vi "UI-Set Dock Button Value.vi"(8 "Error In":errorcluster, 10 "Value (F)":bool, 11 "Appearance Actor in":refnum<class "Appearance Actor.lvclass">) -> (0 "Error Out":errorcluster, 3 "Appearance Actor out":refnum<class "Appearance Actor.lvclass">)   [LabVIEW 2021, in "Appearance Actor.lvlib" / "Appearance Actor.lvclass"]
uses:
  Appearance Actor.lvclass
  Appearance Actor.lvclass/Appearance Actor.ctl
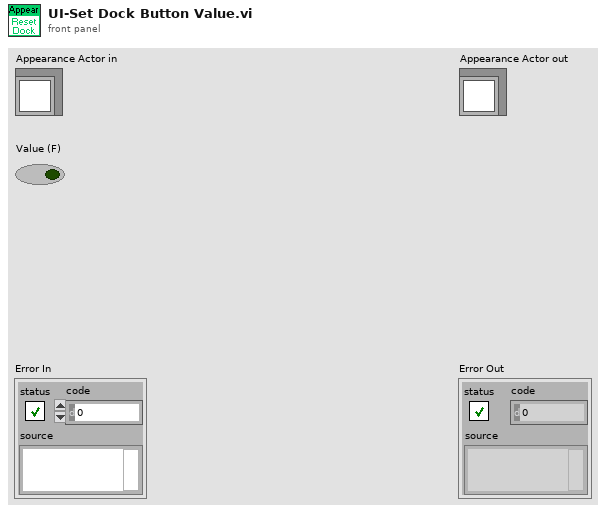
[diagram p1: front panel]
types:
  T1 = typedef "Appearance Actor.lvlib/Appearance Actor.lvclass/UI Controls--map.ctl" = map{string, T2}
  T2 = typedef "Appearance Actor.lvlib/Appearance Actor.lvclass/Element Controls--map.ctl" = map{string, T3}
  T3 = typedef "Appearance Actor.lvlib/Appearance Actor.lvclass/Controls--map.ctl" = map{string, refnum<vi>}
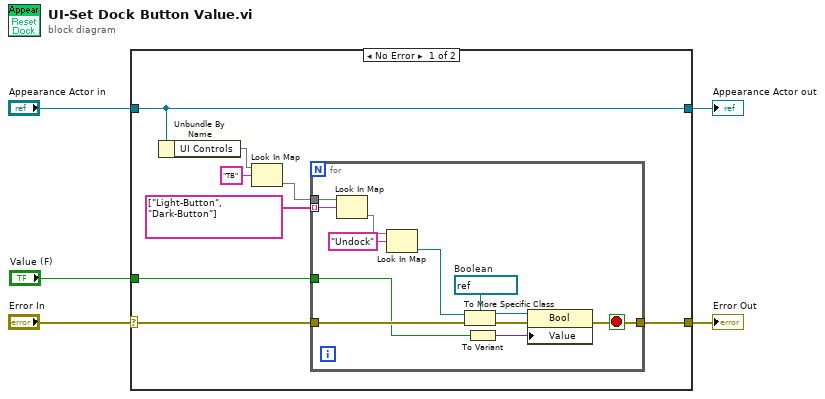
[diagram p0: block diagram]
diagram:
  n1 = case shown="No Error" "Error In" {
    selector: "Error In" -> [w8 w27]
    tunnel: [w7 w27] -> w4
    tunnel: [w13 w26] -> w2
    tunnel: "Appearance Actor in" -> [w13 w26]
    tunnel: "Value (F)" -> [w6 _]
    frame No Error {
      n2 = Unbundle By Name(w13) -> ("UI Controls"=w12:T1)
      n3 = Look In Map(map=w12, key="TB") -> (value=w10:T2)  [unwired: 1 in, 1 out]
      n4 = for {
        tunnel: w10 -> [w25]
        tunnel: string[] ["Light-Button", "Dark-Button"] ("key") -> [w24] mode=indexing
        tunnel: w8 -> [w18]
        tunnel: [w17] -> w7
        tunnel: w6 -> [w15]
        stop <- w17 stop-if-true
        w19 = refnum<vi> refnum  # Boolean
        n5 = Look In Map(map=w25, key=w24) -> (value=w23:T3)  [unwired: 1 in, 1 out]
        n6 = Look In Map(map=w23, key="Undock") -> (value=w16:refnum<vi>)  [unwired: 1 in, 1 out]
        n7 = To More Specific Class(target class=w19, reference=w16, error in=w18) -> (specific class reference=w20:refnum<vi>, error out=w21:errorcluster)
        n8 = To Variant(anything=w15) -> (Variant=w14:variant)
        n9 = property class="Bool"(reference=w20, error in=w21, "Value"=w14) -> (error out=w17:errorcluster)  [unwired: 1 out]
      }
    }
    frame Error {
    }
  }
  "Error Out" <- w4
  "Appearance Actor out" <- w2
